vi "Resize System Rendezvous.vi"(8 "error in (no error)":errorcluster, 9 "New Threads":i32=2, 10 "Rendezvous Index":i32, 11 "System Actor in":refnum<class "System Actor.lvclass">) -> (0 "error out":errorcluster, 3 "System Actor out":refnum<class "System Actor.lvclass">)   [LabVIEW 2024, in "System Actor.lvclass"]
uses:
  System Actor.lvclass
  System Actor.lvclass/System Actor.ctl
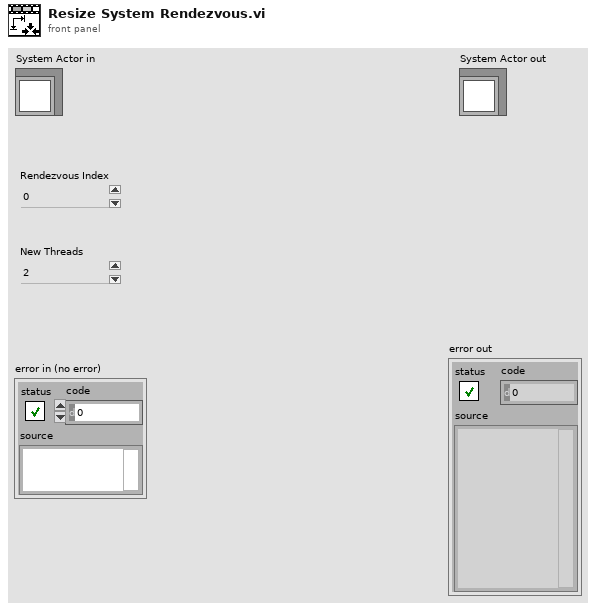
[diagram p1: front panel]
types:
  T1 = typedef "Rendezvous RefNum" = refnum<k1>
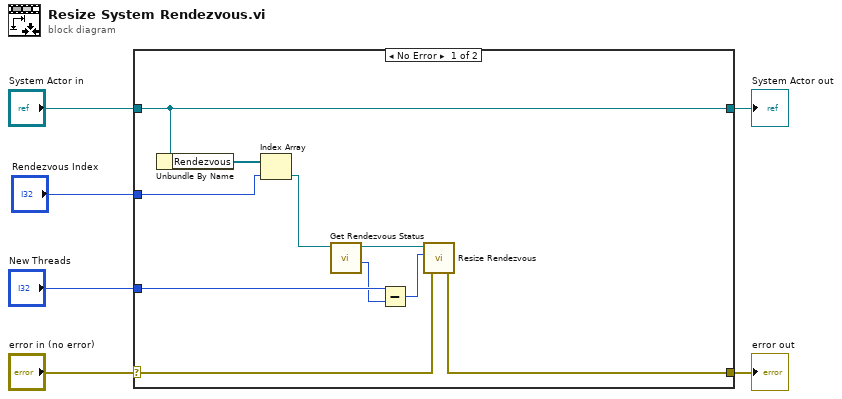
[diagram p0: block diagram]
diagram:
  n1 = case shown="No Error" "error in (no error)" {
    selector: "error in (no error)" -> [w15 w18]
    tunnel: [w16 w18] -> w5
    tunnel: [w14 w17] -> w3
    tunnel: "System Actor in" -> [w14 w17]
    tunnel: "Rendezvous Index" -> [w12 _]
    tunnel: "New Threads" -> [w9 _]
    frame No Error {
      n2 = Unbundle By Name(w14) -> ("Rendezvous"=w13:T1[])
      n3 = Index Array(array=w13, index=w12) -> (element=w11:T1)
      n4 = call <vilib>:"Get Rendezvous Status.vi"("rendezvous"=w11) -> ("size"=w8:i32, "rendezvous out"=w10:T1)  [unwired: 6 in, 3 out]
      n5 = Subtract(x=w9, y=w8) -> (x-y=w7:i32)
      n6 = call <vilib>:"Resize Rendezvous.vi"("error in (no error)"=w15, "size change (0)"=w7, "rendezvous"=w10) -> ("error out"=w16:errorcluster)  [unwired: 2 in, 2 out]
    }
    frame Error {
    }
  }
  "error out" <- w5
  "System Actor out" <- w3
